vi "Add Trace.vi"(5 "Info":string, 7 "LabVIEW Object":refnum<class>, 10 "error in (no error)":errorcluster, 11 "RequestTraceLog in":refnum<class "RequestTraceLog.lvclass">) -> (2 "error out":errorcluster, 3 "RequestTraceLog out":refnum<class "RequestTraceLog.lvclass">)   [LabVIEW 2020, in "HTTP Server.lvlib" / "RequestTraceLog.lvclass"]
uses:
  RequestTraceLog.lvclass
  Trace Item.ctl
  HTTP Server.lvlib
  Processing Step.ctl
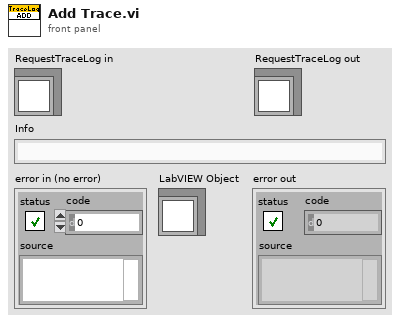
[diagram p1: front panel]
types:
  T1 = typedef "HTTP Server.lvlib/Processing Step.ctl" = enum16{"Connection", "Request", "Routing", "Controller Init", "Controller", "Response", "Complete", "Exception"}
  T2 = typedef "HTTP Server.lvlib/Trace Item.ctl" = cluster{"Duration":dbl, "Step":T1, "Class":string, "Info":string, "Status":bool, "Code":i32, "Time":dbl}
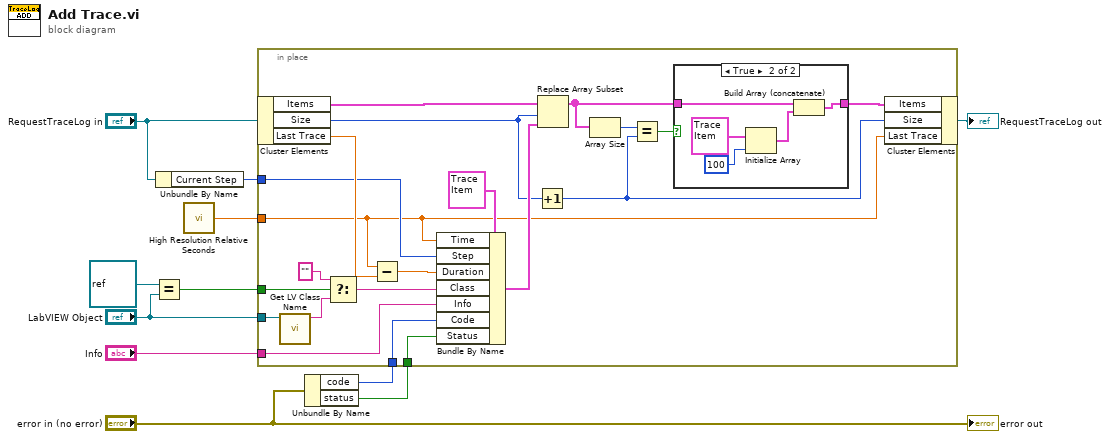
[diagram p0: block diagram]
diagram:
  n1 = Equal?(x=refnum<class> refnum ("LabVIEW Object"), y="LabVIEW Object") -> (x = y?=w5:bool)
  n2 = Unbundle By Name("RequestTraceLog in") -> ("Current Step"=w1:T1)
  n3 = call <vilib>:"High Resolution Relative Seconds.vi"() -> ("relative seconds"=w4:dbl)
  n4 = Unbundle By Name("error in (no error)") -> ("code"=w9:i32, "status"=w3:bool)
  n5 = in-place {
    in-place-border: "LabVIEW Object" -> [w32]
    in-place-border: "Info" -> [w29]
    in-place-border: w9 -> [w28]
    in-place-border: w5 -> [w18]
    in-place-border: w4 -> [w12]
    in-place-border: w3 -> [w15]
    in-place-border: w1 -> [w13]
    n6 = in-place-cluster #1("RequestTraceLog in") -> ("Items"=w27:T2[], "Size"=w25:i32, "Last Trace"=w14:dbl)
    n7 = call <vilib>:"Get LV Class Name.vi"("object"=w32) -> ("class name"=w19:string)  [unwired: 9 in, 1 out]
    n8 = Select(t="", s=w18, f=w19) -> (s? t:f=w16:string)
    n9 = Subtract(x=w12, y=w14) -> (x-y=w30:dbl)
    n10 = Bundle By Name(cluster=T2 {"Duration"=0.0, "Step"=enum."Connection", "Class"="", "Info"="", "Status"=FALSE, "Code"=0, "Time"=0.0} ("Trace Item"), "Time"=w12, "Step"=w13, "Duration"=w30, "Class"=w16, "Info"=w29, "Code"=w28, "Status"=w15) -> (w26:T2)
    n11 = Increment(x=w25) -> (x+1=w23:i32)
    n12 = Replace Array Subset(array=w27, new element=w26, index=w25) -> (w20:T2[])
    n13 = Array Size(array=w20) -> (size(s)=w24:i32)
    n14 = Equal?(x=w24, y=w23) -> (x = y?=w22:bool)
    n15 = case shown="True" w22 {
      tunnel: [w33 w34] -> w21
      tunnel: w20 -> [w33 w36]
      frame False {
      }
      frame True {
        n16 = Initialize Array(T2 {"Duration"=0.0, "Step"=enum."Connection", "Class"="", "Info"="", "Status"=FALSE, "Code"=0, "Time"=0.0} ("Trace Item"), 100 ("dimension size")) -> (w35:T2[])
        n17 = Build Array (concatenate)(w36, w35) -> (w34:T2[])
      }
    }
    n18 = in-place-cluster #1("Items"=w21, "Size"=w23, "Last Trace"=w12) -> (→"RequestTraceLog out":refnum<class "RequestTraceLog.lvclass">)
  }
  "error out" <- "error in (no error)"
